vi "Load Trigger Model Keithley2001 Template.vi"(0 "VISA resource name":refnum<visa-resource-name>, 1 "Arm 1 Bypass":bool=TRUE, 2 "Arm 1 Source":u16(ring) items=["None", "Front Pannel Trigger Key", "Notify Trigger Block 1", "Notify Trigger Block 2", "Notify Trigger Block 3", "Notify Trigger Block 4", "Notify Trigger Block 5", "Notify Trigger Block 6", "Notify Trigger Block 7", "Notify Trigger Block 8", "Command", "Digi IO Line 1", "Digi IO Line 2", "Digi IO Line 3", "Digi IO Line 4", "Digi IO Line 5", "Digi IO Line 6", "TSP-Link 1", "TSP-Link 2", "TSP-Link 3", "LAN 1", "LAN 2", "LAN 3", "LAN 4", "LAN 5", "LAN 6", "LAN 7", "LAN 8", "Blender 1", "Blender 2", "Timer 1", "Timer 2", "Timer 3", "Timer 4", "Analog Trigger", "External Trigger"], 3 "Arm 1 Count":i16=1, 4 "Arm 2 Bypass":bool=TRUE, 5 "Arm 2 Source":u16(ring) items=["None", "Front Pannel Trigger Key", "Notify Trigger Block 1", "Notify Trigger Block 2", "Notify Trigger Block 3", "Notify Trigger Block 4", "Notify Trigger Block 5", "Notify Trigger Block 6", "Notify Trigger Block 7", "Notify Trigger Block 8", "Command", "Digi IO Line 1", "Digi IO Line 2", "Digi IO Line 3", "Digi IO Line 4", "Digi IO Line 5", "Digi IO Line 6", "TSP-Link 1", "TSP-Link 2", "TSP-Link 3", "LAN 1", "LAN 2", "LAN 3", "LAN 4", "LAN 5", "LAN 6", "LAN 7", "LAN 8", "Blender 1", "Blender 2", "Timer 1", "Timer 2", "Timer 3", "Timer 4", "Analog Trigger", "External Trigger"], 6 "Arm 2 Count":i16=1, 7 "error in (no error)":errorcluster, 8 "Arm 2 Delay":dbl, 9 "Trigger Bypass":bool=TRUE, 10 "Trigger Source":u16(ring) items=["None", "Front Pannel Trigger Key", "Notify Trigger Block 1", "Notify Trigger Block 2", "Notify Trigger Block 3", "Notify Trigger Block 4", "Notify Trigger Block 5", "Notify Trigger Block 6", "Notify Trigger Block 7", "Notify Trigger Block 8", "Command", "Digi IO Line 1", "Digi IO Line 2", "Digi IO Line 3", "Digi IO Line 4", "Digi IO Line 5", "Digi IO Line 6", "TSP-Link 1", "TSP-Link 2", "TSP-Link 3", "LAN 1", "LAN 2", "LAN 3", "LAN 4", "LAN 5", "LAN 6", "LAN 7", "LAN 8", "Blender 1", "Blender 2", "Timer 1", "Timer 2", "Timer 3", "Timer 4", "Analog Trigger", "External Trigger"], 11 "Trigger Count":i16=1, 12 "Trigger Delay":dbl) -> (20 "VISA resource name out":refnum<visa-resource-name>, 27 "error Out (no error)":errorcluster)   [LabVIEW 2025, in "Keithley DMM7510.lvlib"]
doc: "This VI loads a predefined trigger model configuration that emulates a Keithley Instruments 2001 trigger model."
uses:
  Keithley DMM7510.lvlib
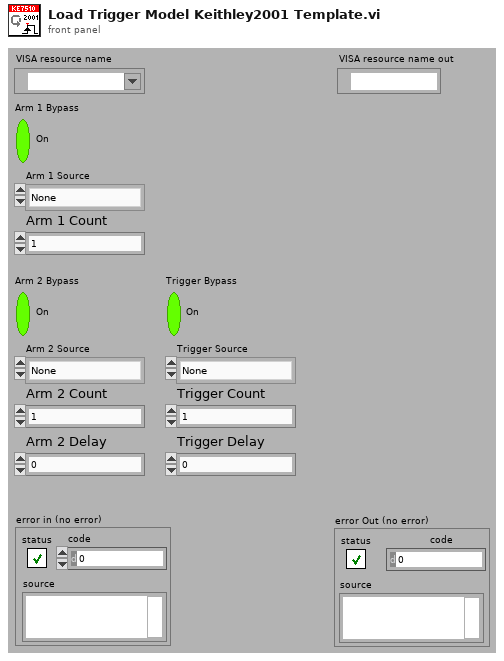
[diagram p1: front panel]
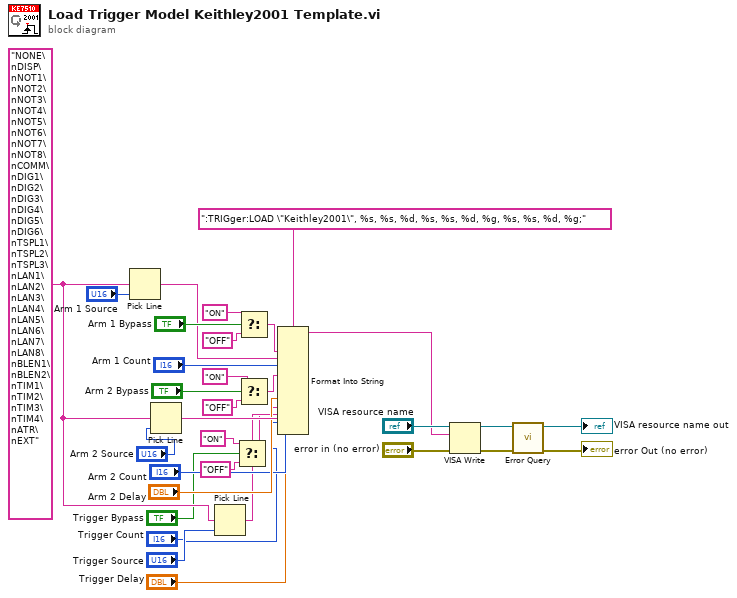
[diagram p0: block diagram]
diagram:
  w9 = "NONE\nDISP\nNOT1\nNOT2\nNOT3\nNOT4\nNOT5\nNOT6\nNOT7\nNOT8\nCOMM\nDIG1\nDIG2\nDIG3\nDIG4\nDIG5\nDIG6\nTSPL1\nTSPL2\nTSPL3\nLAN1\nLAN2\nLAN3\nLAN4\nLAN5\nLAN6\nLAN7\nLAN8\nBLEN1\nBLEN2\nTIM1\nTIM2\nTIM3\nTIM4\nATR\nEXT" ("multi-line string")
  n1 = Pick Line(multi-line string=w9, line index="Arm 1 Source") -> (output string=w19:string)  [unwired: 1 in]
  n2 = Pick Line(multi-line string=w9, line index="Arm 2 Source") -> (output string=w12:string)  [unwired: 1 in]
  n3 = Pick Line(multi-line string=w9, line index="Trigger Source") -> (output string=w7:string)  [unwired: 1 in]
  n4 = Select(t="ON" ("format string"), s="Trigger Bypass", f="OFF" ("format string")) -> (s? t:f=w1:string)
  n5 = Select(t="ON" ("format string"), s="Arm 1 Bypass", f="OFF" ("format string")) -> (s? t:f=w20:string)
  n6 = Select(t="ON" ("format string"), s="Arm 2 Bypass", f="OFF" ("format string")) -> (s? t:f=w14:string)
  n7 = Format Into String(format string=":TRIGger:LOAD \"Keithley2001\", %s, %s, %d, %s, %s, %d, %g, %s, %s, %d, %g;", w20, w19, "Arm 1 Count", w14, w12, "Arm 2 Count", "Arm 2 Delay", w1, w7, "Trigger Count", "Trigger Delay") -> (resulting string=w25:string)  [unwired: 2 in, 1 out]
  n8 = VISA Write(VISA resource name="VISA resource name", write buffer=w25, error in (no error)="error in (no error)") -> (VISA resource name out=w30:refnum<visa-resource-name>, error out=w26:errorcluster)  [unwired: 1 out]
  n9 = call "Error Query.vi"("error in (no error)"=w26, "VISA resource name"=w30) -> ("error out"=→"error Out (no error)":errorcluster, "VISA resource name out"=→"VISA resource name out":refnum<visa-resource-name>)  [unwired: 6 in, 2 out]
